vi "Cannon Set.vi"(0 "Cannon Information":T1) -> ()   [LabVIEW 2012]
uses:
  <vilib>/Rock Robotics/WPI/Solenoid/WPI_SolenoidValue.ctl
  <vilib>/Rock Robotics/WPI/Solenoid/WPI_SolenoidSetEnum.vi
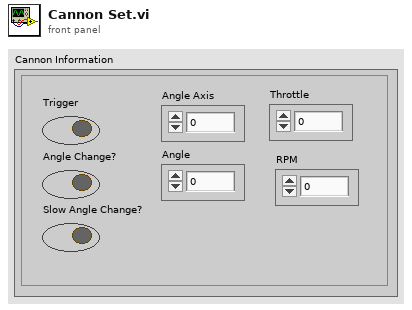
[diagram p1: front panel]
types:
  T1 = cluster{"RPM":dbl, "Trigger":bool, "Angle Axis":dbl, "Angle":dbl, "Throttle":dbl, "Slow Angle Change?":bool, "Angle Change?":bool}
  T2 = typedef "WPI_SolenoidValue.ctl" = enum16{"Off", "On", "Forward", "Reverse"}
  T3 = typedef "WPI_SolenoidDevRef.ctl" = cluster{"DevStatus":errorcluster, "Solenoid Module":T4, "Forward Solenoid Channel":T5, "Reverse Solenoid Channel":T5}
  T4 = typedef "FPGA_TypedefSolenoidModule.ctl" = enum16{"Solenoid Module 1", "Solenoid Module 2"}
  T5 = typedef "WPI_SolenoidChannel.ctl" = enum8{"Solenoid 1", "Solenoid 2", "Solenoid 3", "Solenoid 4", "Solenoid 5", "Solenoid 6", "Solenoid 7", "Solenoid 8", "Invalid"}
  T6 = typedef "WPI_MotorControlDeviceRef.ctl" = cluster{"DeviceStatus":errorcluster, "Type":enum16{"PWM", "CAN"}, "PWM":cluster{"Digital Module":T7, "PWM Channel":T8, "DeadBand":T9}, "CAN":cluster{"Device Number":u8, "Control Mode":T10, "Semaphore":T11, "Max Vout":dbl}, "Invert":bool, "TransformRef":T12, "InvTransformRef":T12}
  T7 = typedef "FPGA_TypedefDigitalModule.ctl" = enum16{"Digital Module 1", "Digital Module 2"}
  T8 = typedef "FPGA_DIOPWMChannel.ctl" = enum8{"PWM 1", "PWM 2", "PWM 3", "PWM 4", "PWM 5", "PWM 6", "PWM 7", "PWM 8", "PWM 9", "PWM 10", "Invalid"}
  T9 = typedef "WPI_PWMDeadband.ctl" = cluster{"Name":string, "maxPositivePwm":i32, "minPositivePwm":i32, "centerPwm":i32, "maxNegativePwm":i32, "minNegativePwm":i32, "angularRange":u16}
  T10 = typedef "WPI_CANJaguar_ControlMode.ctl" = enum8{"Percent VBus", "Current", "Speed", "Position", "Voltage"}
  T11 = typedef "Semaphore RefNum" = refnum<k1>
  T12 = typedef "WPI_PWMTransform_ConPane.ctl" = refnum<vi>
  T13 = typedef "WPI_RelayDevRef.ctl" = cluster{"DevStatus":errorcluster, "Relay Channel":T14, "Digital Module":T7, "Relay Direction":T15}
  T14 = typedef "FPGA_DIORelayChannel.ctl" = enum8{"Relay 1", "Relay 2", "Relay 3", "Relay 4", "Relay 5", "Relay 6", "Relay 7", "Relay 8", "Invalid"}
  T15 = typedef "WPI_RelayDirection.ctl" = enum16{"Both directions", "Forward only", "Reverse only"}
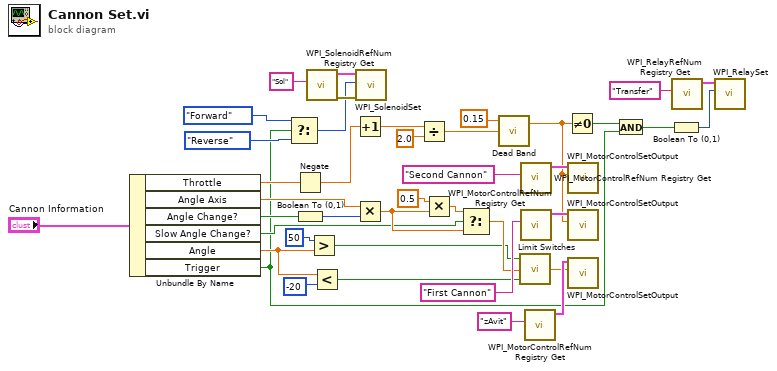
[diagram p0: block diagram]
diagram:
  n1 = Unbundle By Name("Cannon Information") -> ("Throttle"=w30:dbl, "Angle Axis"=w25:dbl, "Angle Change?"=w24:bool, "Slow Angle Change?"=w23:bool, "Angle"=w18:dbl, "Trigger"=w1:bool)
  n2 = Select(t=WPI_SolenoidValue."Forward" ("Value"), s=w1, f=WPI_SolenoidValue."Reverse" ("Value")) -> (s? t:f=w4:T2)
  n3 = Negate(x=w30) -> (-x=w33:dbl)
  n4 = Boolean To (0,1)(Boolean=w24) -> (0, 1=w29:i16)
  n5 = call <vilib>:"WPI_SolenoidRefNum Registry Get.vi"("refnum name"="Sol") -> ("error out"=w6:errorcluster, "SolenoidDevRef"=w3:T3)  [unwired: 9 in]
  n6 = Greater?(x=50, y=w18) -> (0:w15:bool)
  n7 = Less?(x=w18, y=-20) -> (x < y?=w14:bool)
  n8 = Increment(x=w33) -> (x+1=w35:dbl)
  n9 = Multiply(x=w25, y=w29) -> (x*y=w27:dbl)
  n10 = call-poly <vilib>:"WPI_SolenoidSet.vi"("error in (no error)"=w6, "Value"=w4, "SolenoidDevRef"=w3) -> ()  [unwired: 9 out]
  n11 = Divide(x=w35, y=2.0) -> (x/y=w31:dbl)
  n12 = Multiply(x=0.5, y=w27) -> (x*y=w28:dbl)
  n13 = Select(t=w28, s=w23, f=w27) -> (s? t:f=w19:dbl)
  n14 = call "Dead Band.vi"("Axis 1 In"=w31, "Dead Band"=0.15) -> ("Axis 1 Out"=w13:dbl)  [unwired: 1 in, 1 out]
  n15 = call "Limit Switches.vi"("Backward Limit Switch"=w14, "VBus in"=w19, "Forward Limit Switch"=w15) -> ("VBus out"=w20:dbl)
  n16 = call <vilib>:"WPI_MotorControlRefNum Registry Get.vi"("refnum name"="Second Cannon") -> ("MotorControlDevRef"=w38:T6)  [unwired: 9 in, 1 out]
  n17 = call <vilib>:"WPI_MotorControlRefNum Registry Get.vi"("refnum name"="First Cannon") -> ("MotorControlDevRef"=w37:T6)  [unwired: 9 in, 1 out]
  n18 = call <vilib>:"WPI_MotorControlRefNum Registry Get.vi"("refnum name"="zAvit") -> ("MotorControlDevRef"=w21:T6)  [unwired: 9 in, 1 out]
  n19 = Not Equal To 0?(x=w13) -> (x != 0?=w12:bool)
  n20 = call <vilib>:"WPI_MotorControlSetOutput.vi"("Output"=w13, "MotorControlDevRef"=w38) -> ()  [unwired: 7 in, 3 out]
  n21 = call <vilib>:"WPI_MotorControlSetOutput.vi"("Output"=w13, "MotorControlDevRef"=w37) -> ()  [unwired: 7 in, 3 out]
  n22 = call <vilib>:"WPI_MotorControlSetOutput.vi"("Output"=w20, "MotorControlDevRef"=w21) -> ()  [unwired: 7 in, 3 out]
  n23 = And(x=w12, y=w1) -> (x .and. y?=w9:bool)
  n24 = Boolean To (0,1)(Boolean=w9) -> (0, 1=w8:i16)
  n25 = call <vilib>:"WPI_RelayRefNum Registry Get.vi"("refnum name"="Transfer") -> ("RelayDevRef"=w10:T13)  [unwired: 9 in, 1 out]
  n26 = call <vilib>:"WPI_RelaySet.vi"("RelayValue"=w8, "RelayDevRef"=w10) -> ()  [unwired: 8 in, 2 out]
